vi "Determine Current Pose.vi"(7 "Wrist HW":T8, 10 "Extend HW":T7, 11 "Sholder HW":T1) -> (3 "Current Pose Out":T9)   [LabVIEW 2020, in "MotionMaster_SubCMD.lvlib"]
uses:
  MotionMaster_SubCMD.lvlib
  Shared Code/TypeDefs/Cluster_Pose Positions.ctl
  Shared Code/TypeDefs/Cluster_FX Sensor Values.ctl
  Shared Code/TypeDefs/Cluster_FX CloseLoop Values.ctl
  Shared Code/TypeDefs/Cluster_FX Limit Switchs.ctl
  Shared Code/TypeDefs/Cluster_FX Current Values.ctl
  Shared Code/TypeDefs/Cluster_FX Integrated Sensor Values.ctl
  Shared Code/TypeDefs/Cluster_Wrist HW Outputs.ctl
  Shared Code/TypeDefs/Cluster_Extend HW Outputs.ctl
  Shared Code/TypeDefs/Cluster_Sholder_HW Outputs.ctl
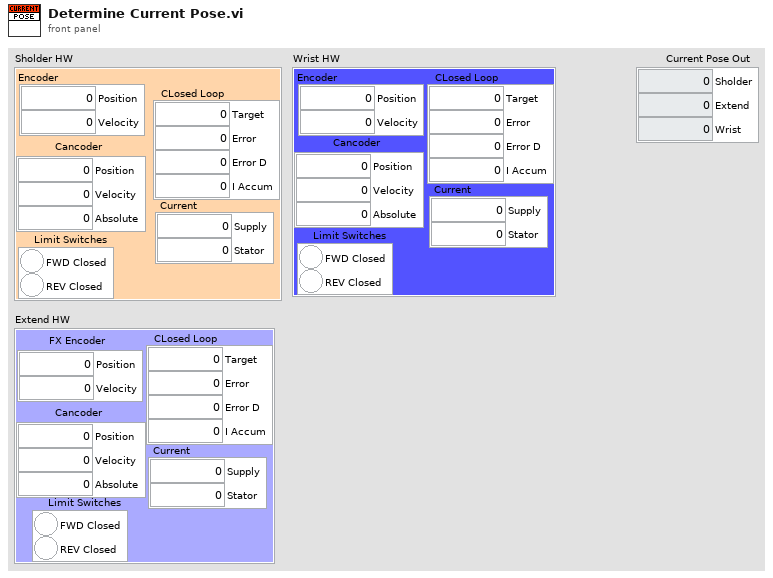
[diagram p1: front panel]
types:
  T1 = typedef "Cluster_Sholder_HW Outputs.ctl" = cluster{"Encoder":T2, "CLosed Loop":T3, "Limit Switches":T4, "Current":T5, "Cancoder":T6}
  T2 = typedef "Cluster_FX Sensor Values.ctl" = cluster{"Position":i32, "Velocity":i32}
  T3 = typedef "Cluster_FX CloseLoop Values.ctl" = cluster{"Target":dbl, "Error":i32, "Error D":dbl, "I Accum":dbl}
  T4 = typedef "Cluster_FX Limit Switchs.ctl" = cluster{"FWD Closed":bool, "REV Closed":bool}
  T5 = typedef "Cluster_FX Current Values.ctl" = cluster{"Supply":dbl, "Stator":dbl}
  T6 = typedef "Cluster_FX Integrated Sensor Values.ctl" = cluster{"Position":dbl, "Velocity":dbl, "Absolute":dbl}
  T7 = typedef "Cluster_Extend HW Outputs.ctl" = cluster{"CLosed Loop":T3, "Limit Switches":T4, "Current":T5, "FX Encoder":T2, "Cancoder":T6}
  T8 = typedef "Cluster_Wrist HW Outputs.ctl" = cluster{"Encoder":T2, "CLosed Loop":T3, "Limit Switches":T4, "Current":T5, "Cancoder":T6}
  T9 = typedef "Cluster_Pose Positions.ctl" = cluster{"Sholder":i32, "Extend":i32, "Wrist":i32}
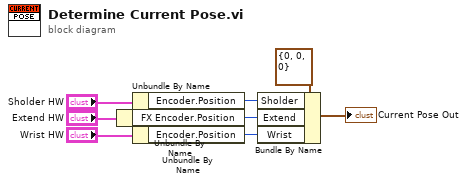
[diagram p0: block diagram]
diagram:
  n1 = Unbundle By Name("Extend HW") -> ("FX Encoder.Position"=w2:i32)
  n2 = Unbundle By Name("Sholder HW") -> ("Encoder.Position"=w3:i32)
  n3 = Unbundle By Name("Wrist HW") -> ("Encoder.Position"=w1:i32)
  n4 = Bundle By Name(cluster=T9 {"Sholder"=0, "Extend"=0, "Wrist"=0} ("Current Pose"), "Sholder"=w3, "Extend"=w2, "Wrist"=w1) -> (→"Current Pose Out":T9)
